vi "FindEnumValues.vi"(11 "string":string) -> (1 "PropertyFound":bool, 3 "properties":T1)   [LabVIEW 2013, in "CS.lvclass"]
uses:
  CS.lvclass
  baseClass/propertyDef.ctl
  baseClass/types.ctl
  baseClass/baseClass.lvclass
panel:
  out "match + rest of string":string
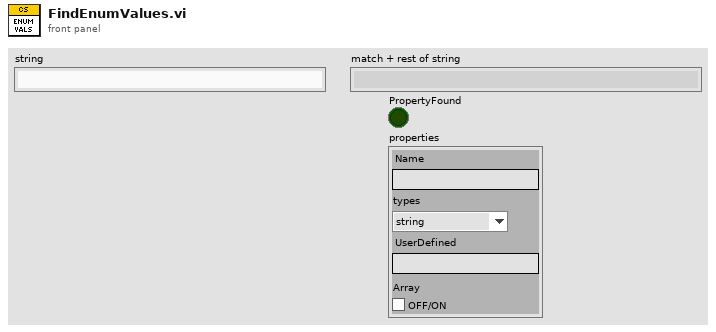
[diagram p1: front panel]
types:
  T1 = typedef "baseClass.lvclass/propertyDef.ctl" = cluster{"Name":string, "types":T2, "UserDefined":string, "Array":bool}
  T2 = typedef "baseClass.lvclass/types.ctl" = enum16{"string", "int", "decimal", "bool", "class", "enum"}
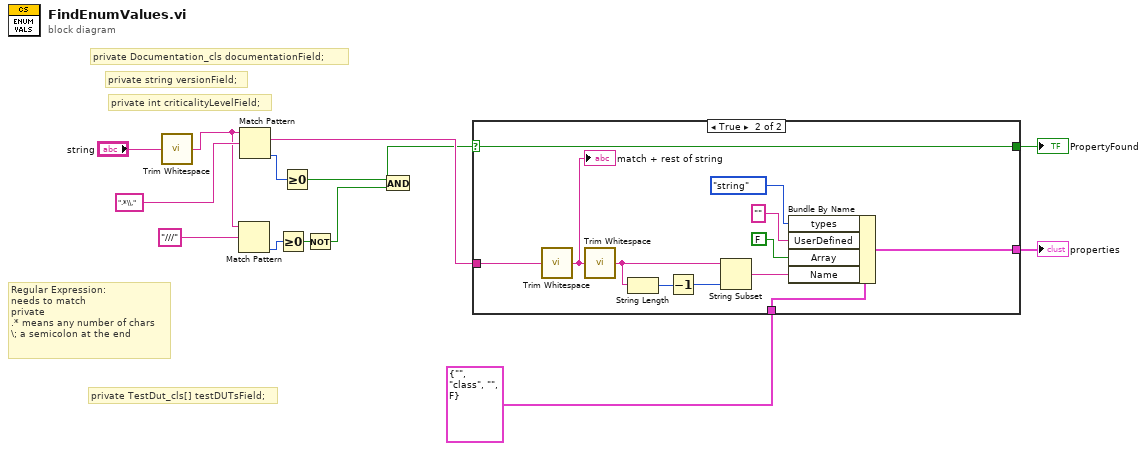
[diagram p0: block diagram]
diagram:
  # "private TestDut_cls[] testDUTsField;"
  # "Regular Expression:\nneeds to match\nprivate\n.* means any number of chars\n\\; a semicolon at the end"
  # "private int criticalityLevelField;"
  # "private string versionField;"
  # "private Documentation_cls documentationField;"
  n1 = call <vilib>:"Trim Whitespace.vi"("string"="string") -> ("trimmed string"=w7:string)  [unwired: 1 in]
  n2 = Match Pattern(string=w7, regular expression="///") -> (offset past match=w5:i32)  [unwired: 1 in, 3 out]
  n3 = Match Pattern(string=w7, regular expression=".*\\,") -> (match substring=w11:string, offset past match=w12:i32)  [unwired: 1 in, 2 out]
  n4 = Greater Or Equal To 0?(x=w5) -> (x >= 0?=w4:bool)
  n5 = Greater Or Equal To 0?(x=w12) -> (x >= 0?=w2:bool)
  n6 = Not(x=w4) -> (.not. x?=w3:bool)
  n7 = And(x=w2, y=w3) -> (x .and. y?=w1:bool)
  n8 = case shown="True" w1 {
    selector: w1 -> [_ w23]
    tunnel: w11 -> [_ w20]
    tunnel: [_ w23] -> w10
    tunnel: T1 {"Name"="", "types"=enum."class", "UserDefined"="", "Array"=FALSE} ("properties") -> [_ w22]
    tunnel: [_ w21] -> w8
    frame False {
    }
    frame True {
      n9 = call <vilib>:"Trim Whitespace.vi"("string"=w20) -> ("trimmed string"=w17:string)  [unwired: 1 in]
      "match + rest of string" <- w17
      n10 = call <vilib>:"Trim Whitespace.vi"("string"=w17) -> ("trimmed string"=w26:string)  [unwired: 1 in]
      n11 = String Length(string=w26) -> (length=w25:i32)
      n12 = Decrement(x=w25) -> (x-1=w24:i32)
      n13 = String Subset(string=w26, length (rest)=w24) -> (substring=w19:string)  [unwired: 1 in]
      n14 = Bundle By Name(cluster=w22, "types"=types."string", "UserDefined"="", "Array"=FALSE, "Name"=w19) -> (w21:T1)
    }
  }
  "PropertyFound" <- w10
  "properties" <- w8
